vi "Euclidean Distance VI.vi"(8 "Reference":dbl[](array[numeric]), 11 "Test":dbl[](array[numeric])) -> (2 "Dist":dbl)   [LabVIEW 2012]
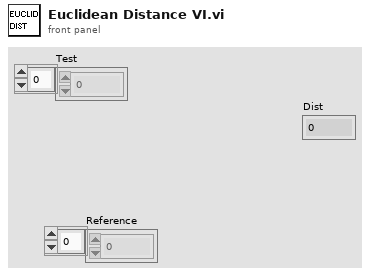
[diagram p1: front panel]
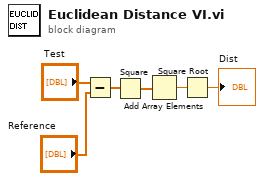
[diagram p0: block diagram]
diagram:
  n1 = Subtract(x="Test", y="Reference") -> (x-y=w5:dbl[])
  n2 = Square(x=w5) -> (x^2=w4:dbl[])
  n3 = Add Array Elements(numeric array=w4) -> (sum=w3:dbl)
  n4 = Square Root(x=w3) -> (sqrt(x)=→"Dist":dbl)
